vi "Decode enum.vi"(10 "Wire Type":T1, 11 "Data":u8[](array[numeric]) format="%.0x") -> (2 "error out":errorcluster, 3 "Enumeration":T2)   [LabVIEW 2020, in "ServiceType.lvlib"]
uses:
  ServiceType.lvlib
  Enumeration.ctl
  lv-protoc/LV-Proto/Wire Type.ctl
  lv-protoc/LV-Proto/LV-Proto.lvlib
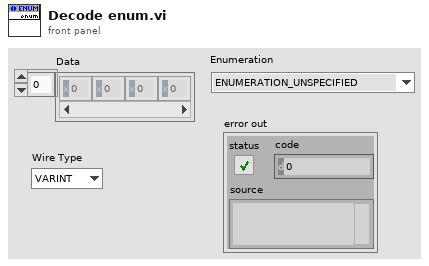
[diagram p1: front panel]
types:
  T1 = typedef "LV-Proto.lvlib/Wire Type.ctl" = enum8{"VARINT", "I64", "LEN", "SGROUP (Deprecated)", "EGROUP (Deprecated)", "I32"}
  T2 = typedef "ServiceType.lvlib/Enumeration.ctl" = enum16{"ENUMERATION_UNSPECIFIED"}
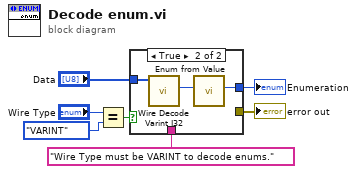
[diagram p0: block diagram]
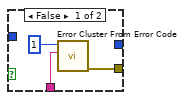
[diagram p2: hidden frame]
diagram:
  n1 = Equal?(x="Wire Type", y=Wire_Type."VARINT") -> (x = y?=w7:bool)
  n2 = case shown="True" w7 {
    tunnel: "Data" -> [_ w13]
    tunnel: [w9 _] -> w1
    tunnel: "Wire Type must be VARINT to decode enums." -> [w8 _]
    tunnel: [_ w11] -> w2
    frame False {
      n3 = call <vilib>:"Error Cluster From Error Code.vi"("error message (\"\")"=w8, "error code (0)"=1) -> ("error out"=w9:errorcluster)  [unwired: 7 in]
    }
    frame True {
      n4 = call "Wire Decode Varint I32.vi"("Buffer in"=w13) -> ("I32"=w12:i32)  [unwired: 9 in, 1 out]
      n5 = call "Enum from Value.vi"("Value"=w12) -> ("Enumeration"=w11:T2)  [unwired: 10 in]
    }
  }
  "Enumeration" <- w2
  "error out" <- w1
